vi "Init_UI_Stop.vi"(8 "error in (no error)":errorcluster, 11 "Cluster_IN":T1) -> (0 "error out":errorcluster, 3 "Cluster_OUT":T1)   [LabVIEW 2020]
uses:
  Controls/UI_Cluster.ctl
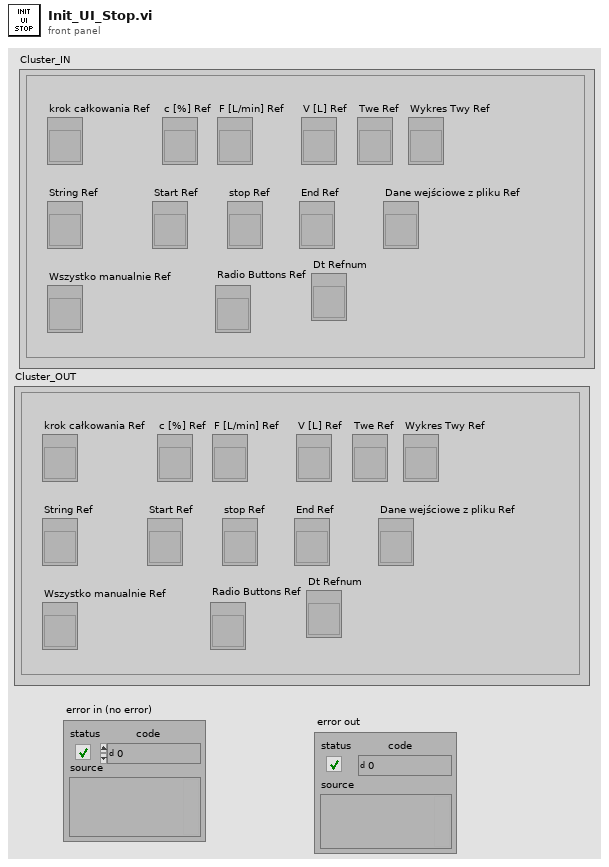
[diagram p1: front panel]
types:
  T1 = typedef "UI_Cluster.ctl" = cluster{"krok całkowania Ref":refnum<vi>, "c [%] Ref":refnum<vi>, "F [L/min] Ref":refnum<vi>, "V [L] Ref":refnum<vi>, "Twe Ref":refnum<vi>, "Wykres Twy Ref":refnum<vi>, "String Ref":refnum<vi>, "Start Ref":refnum<vi>, "stop Ref":refnum<vi>, "End Ref":refnum<vi>, "Dane wejściowe z pliku Ref":refnum<vi>, "Wszystko manualnie Ref":refnum<vi>, "Dt Refnum":refnum<vi>, "Radio Buttons Ref":refnum<vi>}
  T2 = enum8{"Enabled", "Disabled", "Disabled and Grayed Out"}
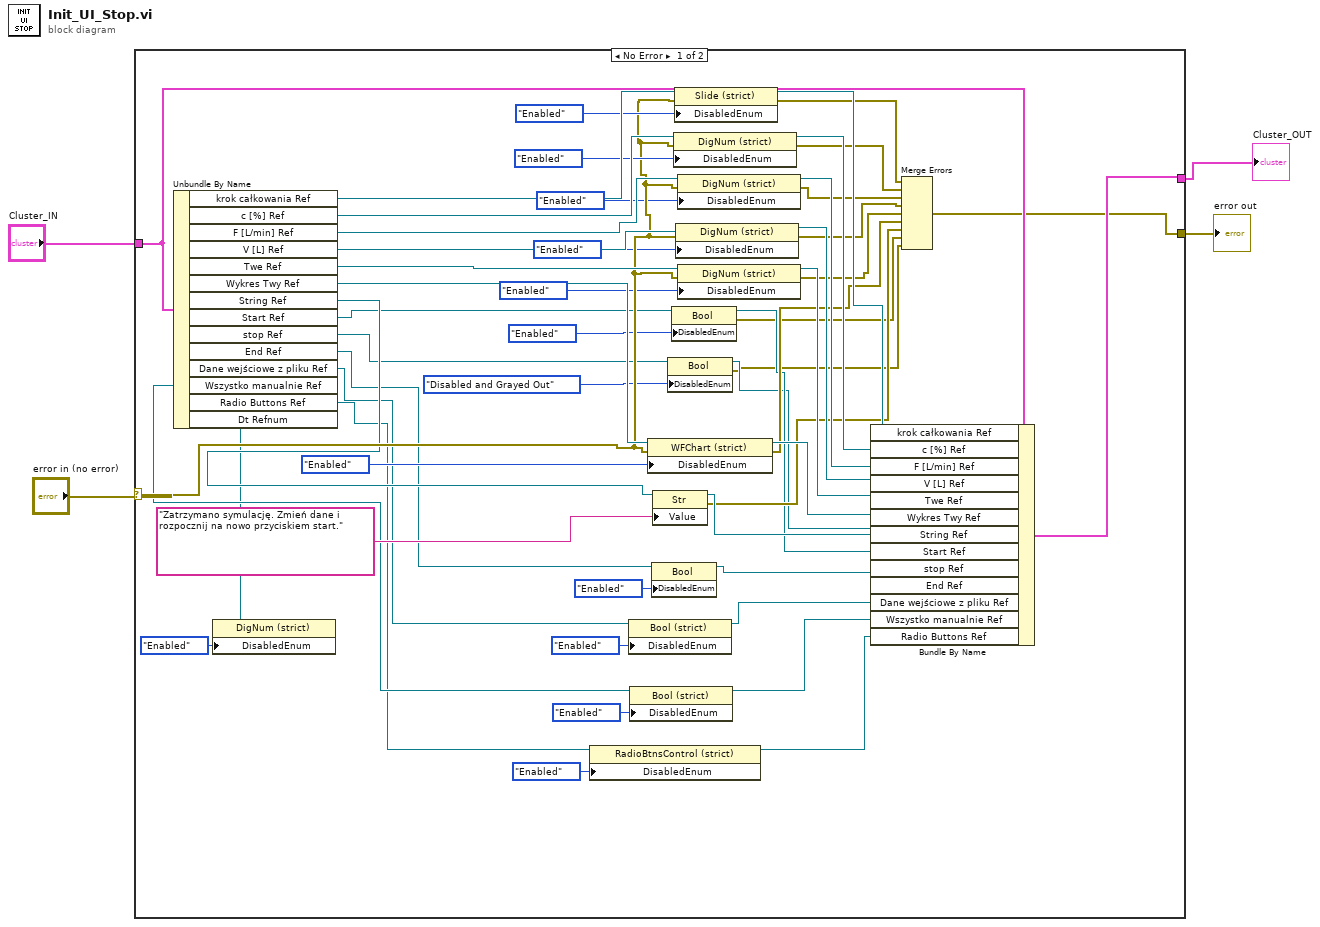
[diagram p0: block diagram]
diagram:
  n1 = case shown="No Error" "error in (no error)" {
    selector: "error in (no error)" -> [w41 w59]
    tunnel: "Cluster_IN" -> [w52 w60]
    tunnel: [w42 w60] -> w2
    tunnel: [w34 w59] -> w1
    frame No Error {
      n2 = Unbundle By Name(w52) -> ("krok całkowania Ref"=w58:refnum<vi>, "c [%] Ref"=w56:refnum<vi>, "F [L/min] Ref"=w49:refnum<vi>, "V [L] Ref"=w54:refnum<vi>, "Twe Ref"=w53:refnum<vi>, "Wykres Twy Ref"=w45:refnum<vi>, "String Ref"=w33:refnum<vi>, "Start Ref"=w27:refnum<vi>, "stop Ref"=w26:refnum<vi>, "End Ref"=w18:refnum<vi>, "Dane wejściowe z pliku Ref"=w15:refnum<vi>, "Wszystko manualnie Ref"=w14:refnum<vi>, "Radio Buttons Ref"=w9:refnum<vi>, "Dt Refnum"=w6:refnum<vi>)
      n3 = property class="DigNum (strict)"(reference=w6, "DisabledEnum"=T2."Enabled" ("Disabled")) -> ()  [unwired: 1 in, 2 out]
      n4 = property class="RadioBtnsControl (strict)"(reference=w9, "DisabledEnum"=T2."Enabled" ("Disabled")) -> (reference out=w7:refnum<vi>)  [unwired: 1 in, 1 out]
      n5 = property class="Bool (strict)"(reference=w15, "DisabledEnum"=T2."Enabled" ("Disabled")) -> (reference out=w11:refnum<vi>)  [unwired: 1 in, 1 out]
      n6 = property class="Bool (strict)"(reference=w14, "DisabledEnum"=T2."Enabled" ("Disabled")) -> (reference out=w10:refnum<vi>)  [unwired: 1 in, 1 out]
      n7 = property class="WFChart (strict)"(reference=w45, error in=w41, "DisabledEnum"=T2."Enabled" ("Disabled")) -> (reference out=w43:refnum<vi>, error out=w35:errorcluster)
      n8 = property class="Bool"(reference=w18, "DisabledEnum"=T2."Enabled" ("Disabled")) -> (reference out=w16:refnum<vi>)  [unwired: 1 in, 1 out]
      n9 = property class="Str"(reference=w33, "Value"="Zatrzymano symulację. Zmień dane i rozpocznij na nowo przyciskiem start.") -> (reference out=w31:refnum<vi>, error out=w23:errorcluster)  [unwired: 1 in]
      n10 = property class="Bool"(reference=w26, "DisabledEnum"=T2."Disabled and Grayed Out" ("Disabled")) -> (reference out=w21:refnum<vi>, error out=w19:errorcluster)  [unwired: 1 in]
      n11 = property class="Bool"(reference=w27, "DisabledEnum"=T2."Enabled" ("Disabled")) -> (reference out=w22:refnum<vi>, error out=w20:errorcluster)  [unwired: 1 in]
      n12 = property class="DigNum (strict)"(reference=w56, error in=w41, "DisabledEnum"=T2."Enabled" ("Disabled")) -> (reference out=w50:refnum<vi>, error out=w39:errorcluster)
      n13 = property class="Slide (strict)"(reference=w58, error in=w41, "DisabledEnum"=T2."Enabled" ("Disabled")) -> (reference out=w51:refnum<vi>, error out=w40:errorcluster)
      n14 = property class="DigNum (strict)"(reference=w54, error in=w41, "DisabledEnum"=T2."Enabled" ("Disabled")) -> (reference out=w47:refnum<vi>, error out=w37:errorcluster)
      n15 = property class="DigNum (strict)"(reference=w49, error in=w41, "DisabledEnum"=T2."Enabled" ("Disabled")) -> (reference out=w48:refnum<vi>, error out=w38:errorcluster)
      n16 = property class="DigNum (strict)"(reference=w53, error in=w41, "DisabledEnum"=T2."Enabled" ("Disabled")) -> (reference out=w46:refnum<vi>, error out=w36:errorcluster)
      n17 = Bundle By Name(cluster=w52, "krok całkowania Ref"=w51, "c [%] Ref"=w50, "F [L/min] Ref"=w48, "V [L] Ref"=w47, "Twe Ref"=w46, "Wykres Twy Ref"=w43, "String Ref"=w31, "Start Ref"=w22, "stop Ref"=w21, "End Ref"=w16, "Dane wejściowe z pliku Ref"=w11, "Wszystko manualnie Ref"=w10, "Radio Buttons Ref"=w7) -> (w42:T1)
      n18 = Merge Errors(w40, w39, w38, w37, w36, w35, w23, w20, w19) -> (w34:errorcluster)
    }
    frame Error {
    }
  }
  "Cluster_OUT" <- w2
  "error out" <- w1
